vi "Actor Core.vi"(8 "error in":errorcluster, 11 "Example Controller":refnum<class "Example Controller.lvclass">) -> (0 "error out":errorcluster, 3 "Actor out":refnum<class "Actor.lvclass">)   [LabVIEW 2023, in "Example MVC Actors.lvlib" / "Example Controller.lvlib" / "Example Controller.lvclass"]
doc: "This is Actor Core.vi, the main message handling loop for Actors. An actor usually just sits in this loop and processes messages as they arrive. Any error returned by the message Do.vi call will stop the loop, with error code 43 as the cannonical signal to stop with no error sent to caller. Descendants may override that in Handle Error.vi."
uses:
  Example Controller.lvclass
  <vilib>/ActorFramework/Actor/Actor.lvclass
  Registered Views.ctl
  Controller/View Settings.ctl
  Example Controller.lvclass/Example Controller.ctl
  Controller/Controller.lvclass/Controller.ctl
  <vilib>/ActorFramework/Actor/Actor.lvclass/Actor.ctl
  <vilib>/ActorFramework/Message Enqueuer/Message Enqueuer.lvclass/Message Enqueuer.ctl
  Write Boolean Notifier.vi
  Controller/properties/Read Registered Views Event Ref.vi
  Controller/properties/Read View Settings Event Ref.vi
  <vilib>/ActorFramework/Message Enqueuer/Init from Existing Queue.vi
  <vilib>/ActorFramework/Message Enqueuer/Enqueue.vi
  <vilib>/ActorFramework/Stop Msg/Stop Msg.lvclass
  <vilib>/Utility/LVClass/Get LV Class Name.vi
  <resource>/AFDebug/Generate Trace for Message.vi
  <vilib>/ActorFramework/Message Priority Queue/Priority Enqueue.vi
  <vilib>/ActorFramework/Message Enqueuer/Message Enqueuer.lvclass
  Timed Loop Controller/Timed Loop Controller/Timed Loop Controller.lvclass
  Controller/Controller.lvclass
  Controller Messages/Read View Settings Msg/Read View Settings Msg.lvclass
  Controller Messages/Write View Settings Msg/Write View Settings Msg.lvclass
  <userlib>/_OpenG.lib/error/error.llb/openg_error.lvlib
  Example Controller Messages/Launch Feature Test View Msg/Launch Feature Test View Msg.lvclass
panel:
  in  "Launch  Feature Test View":bool
  in  "View Settings":T1
  in  "Write View Settings":bool
  in  "Read View Settings":bool
  out "View Settings Read":T1
  in  "View":T2
  out "Boolean Chart":i16(graph)
  in  "Stop Button":bool
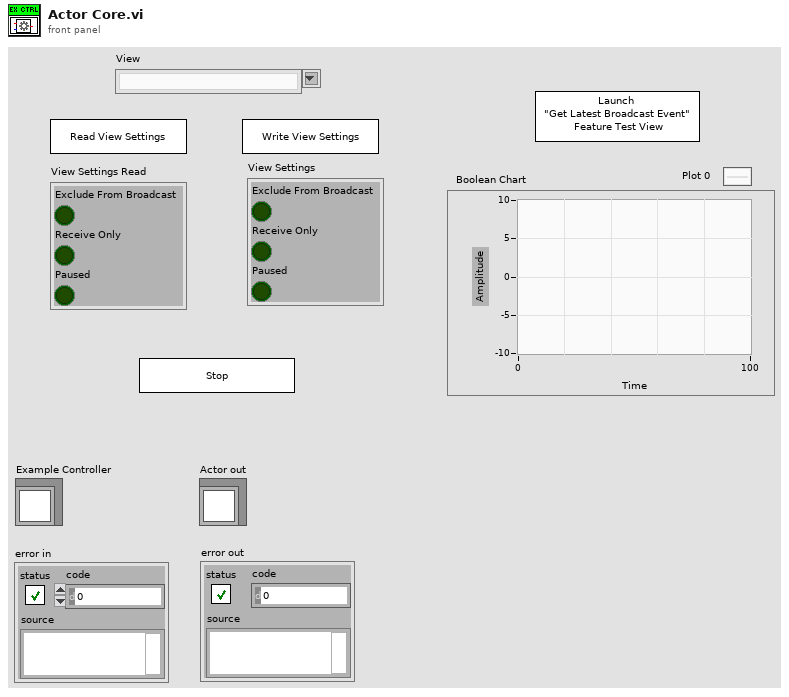
[diagram p1: front panel]
types:
  T1 = typedef "MVC Actors.lvlib/Controller.lvclass/View Settings.ctl" = cluster{"Exclude From Broadcast":bool, "Receive Only":bool, "Paused":bool}
  T2 = typedef "Example MVC Actors.lvlib/Example Controller.lvlib/Example Controller.lvclass/Registered Views.ctl" = string
  T3 = enum8{"Enabled", "Disabled", "Disabled and Grayed Out"}
  T4 = typedef "MVC Actors.lvlib/Controller.lvclass/Registered Views Event Ref.ctl" = refnum<user-event>
  T5 = typedef "MVC Actors.lvlib/Controller.lvclass/View Settings Event Ref.ctl" = refnum<user-event>
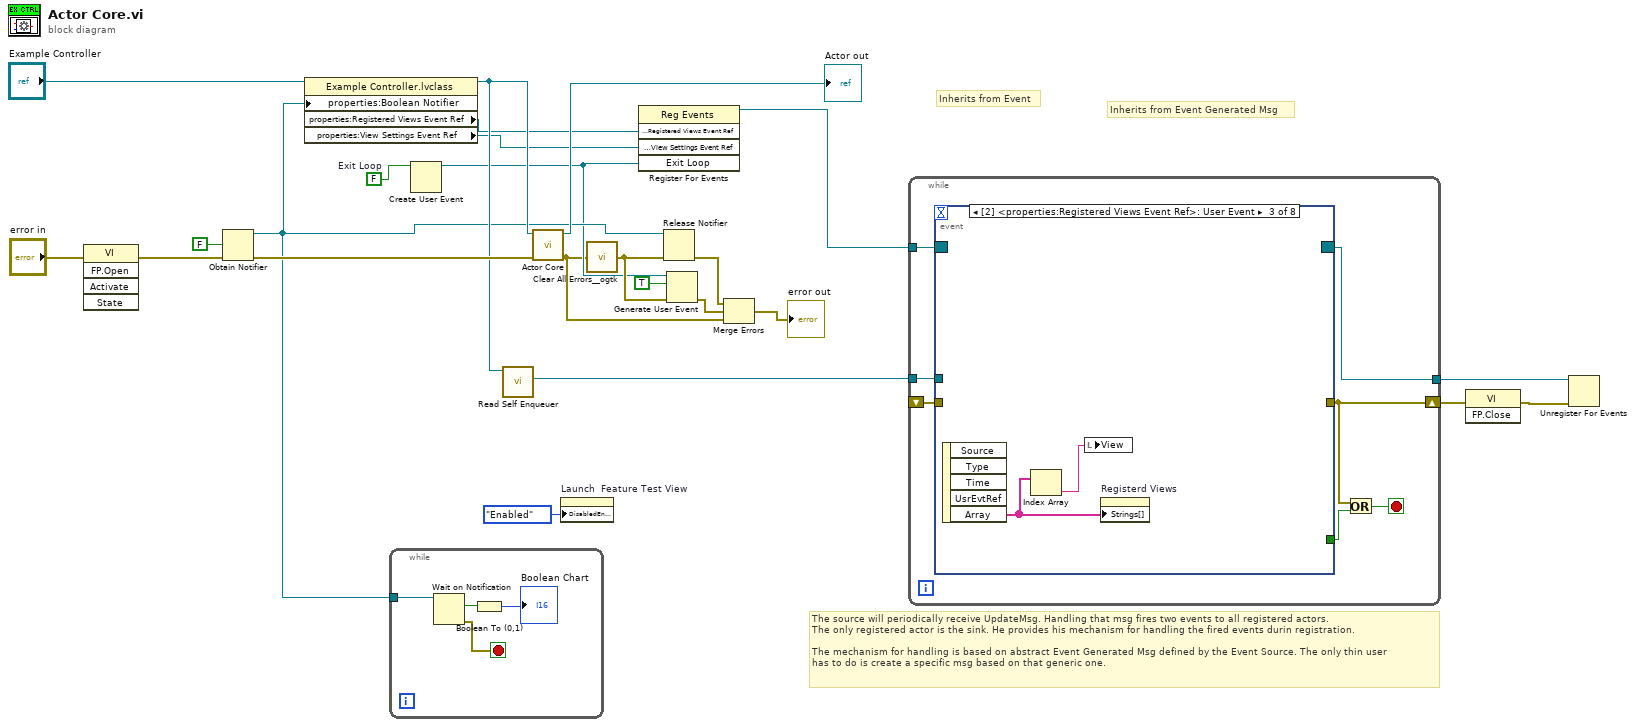
[diagram p0: block diagram]
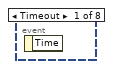
[diagram p2: hidden frame]
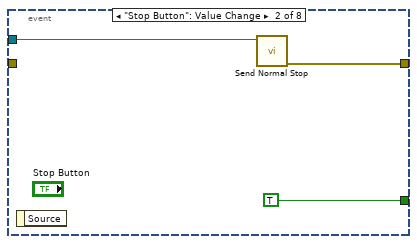
[diagram p3: hidden frame]
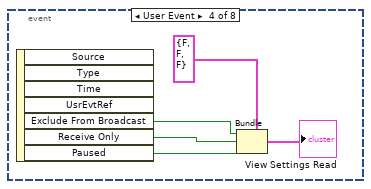
[diagram p4: hidden frame]
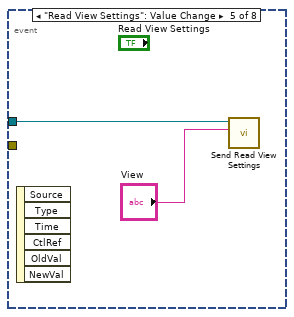
[diagram p5: hidden frame]
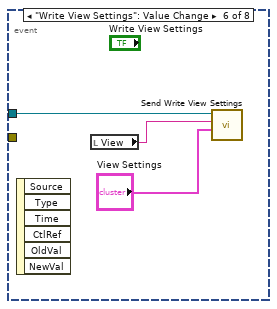
[diagram p6: hidden frame]
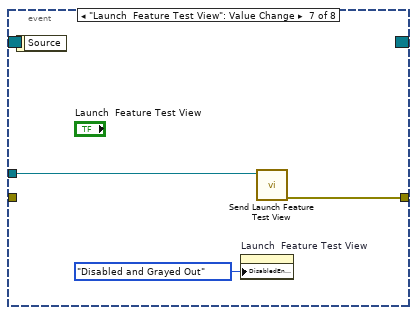
[diagram p7: hidden frame]
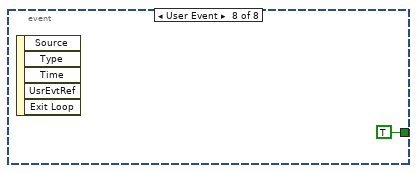
[diagram p8: hidden frame]
diagram:
  w11 = FALSE  # Exit Loop
  # "The source will periodically receive UpdateMsg. Handling that msg fires two events to all registered actors.\nThe only registered actor is the sink. He provides his mechanism for handling the fired events durin registration.\n\nThe mechanism for handling is based on abstract Event Generated Msg defined by the Event Source. The only thin user\nhas to do is create a specific msg based on that generic one."
  # "Inherits from Event"
  # "Inherits from Event Generated Msg"
  n1 = invoke on="Invoke Node" class="VI" method="FP.Open"(error in="error in") -> (error out=w2:errorcluster)  [unwired: 4 in, 4 out]
  n2 = Obtain Notifier(notification data type=FALSE, error in (no error)=w2) -> (notifier out=w18:refnum<notifier>, error out=w20:errorcluster)  [unwired: 2 in, 1 out]
  n3 = property class="Example Controller.lvclass"(reference="Example Controller", "properties:Boolean Notifier"=w18) -> (reference out=w19:refnum<class "Example Controller.lvclass">, "properties:Registered Views Event Ref"=w17:T4, "properties:View Settings Event Ref"=w16:T5)  [unwired: 1 in, 1 out]
  n4 = while {
    tunnel: w18 -> [w28]
    stop <- w25 stop-if-true
    n5 = Wait on Notification(notifier=w28) -> (notification=w27:bool, error out=w25:errorcluster)  [unwired: 3 in, 2 out]
    n6 = Boolean To (0,1)(Boolean=w27) -> (0, 1=→"Boolean Chart":i16)
  }
  n7 = Create User Event(user event datatype=w11) -> (user event=w8:refnum<user-event>)  [unwired: 1 in, 1 out]
  n8 = call <vilib>:"Read Self Enqueuer.vi"("Actor"=w19) -> ("Self Enqueuer"=w12:refnum<class "Message Enqueuer.lvclass">)  [unwired: 10 in]
  n9 = call-parent "Actor Core.vi"("error in"=w20, "Timed Loop Controller"=w19) -> ("error out"=w5:errorcluster, "Actor out"=→"Actor out":refnum<class "Actor.lvclass">)  [unwired: 8 in]
  n10 = property on="Launch  Feature Test View" class="Bool"("DisabledEnum"=T3."Enabled" ("Disabled")) -> ()  [unwired: 2 in, 2 out]
  n11 = call <userlib>:"Clear All Errors__ogtk.vi"("Error In"=w5) -> ("Error Out"=w9:errorcluster)  [unwired: 3 in]
  n12 = register-events(w17, w16, w8) -> (reference out=w15:refnum<event-registration>)  [unwired: 2 in, 1 out]
  n13 = Release Notifier(notifier=w18, error in (no error)=w9) -> (error out=w7:errorcluster)  [unwired: 1 in, 2 out]
  n14 = Generate User Event(user event=w8, event data cluster=TRUE ("event data"), error in=w9) -> (error out=w6:errorcluster)  [unwired: 1 in, 1 out]
  n15 = Merge Errors(w7, w6, w5) -> (→"error out":errorcluster)
  n16 = while {
    tunnel: w12 -> [w34]
    shift-right: [w32] -> w23
    shift-left: _ -> [w35]
    tunnel: w15 -> [w30]
    tunnel: [w29] -> w13
    stop <- w31 stop-if-true
    n17 = event shown="[2] <properties:Registered Views Event Ref>: User Event" {
      selector: w30 -> [_ _ _ _ _ _ _ _]
      dyn-events: [_ _ _ _ _ _ _ _] -> w29
      timeout: _ -> [_ _ _ _ _ _ _ _]
      tunnel: w35 -> [_ _ _ _ _ _ _ _]
      tunnel: w34 -> [_ w37 _ _ w46 w48 w53 _]
      tunnel: [_ w38 _ _ _ _ w52 _] -> w32
      tunnel: [_ TRUE _ _ _ _ _ TRUE] -> w33
      event Timeout {
        n18 = event-data() -> ()  [unwired: 1 in, 1 out]
      }
      event "Stop Button": Value Change {
        n19 = event-data() -> ()  [unwired: 1 in, 1 out]
        n20 = call <vilib>:"Send Normal Stop.vi"("Message Enqueuer"=w37) -> ("error out"=w38:errorcluster)  [unwired: 10 in]
      }
      event User Event {
        n21 = event-data() -> ("Array"=w40:string[])  [unwired: 1 in, 4 out]
        n22 = Index Array(array=w40) -> (element=w39:string)  [unwired: 1 in]
        n23 = local write "View"(w39) -> ()
        n24 = property on="Registerd Views" class="CmbBox (strict)"("Strings[]"=w40) -> ()  [unwired: 2 in, 2 out]
      }
      event User Event {
        n25 = event-data() -> ("Exclude From Broadcast"=w44:bool, "Receive Only"=w43:bool, "Paused"=w42:bool)  [unwired: 1 in, 4 out]
        n26 = Bundle(cluster=T1 {"Exclude From Broadcast"=FALSE, "Receive Only"=FALSE, "Paused"=FALSE} ("Sink Settings"), "Exclude From Broadcast"=w44, "Receive Only"=w43, "Paused"=w42) -> (→"View Settings Read":T1)
      }
      event "Read View Settings": Value Change {
        n27 = event-data() -> ()  [unwired: 1 in, 6 out]
        n28 = call "Send Read View Settings.vi"("View Name"="View", "Message Enqueuer in"=w46) -> ()  [unwired: 8 in, 2 out]
      }
      event "Write View Settings": Value Change {
        n29 = event-data() -> ()  [unwired: 1 in, 6 out]
        n30 = local read "View"() -> (w49:T2)
        n31 = call "Send Write View Settings.vi"("View Settings"="View Settings", "View Name"=w49, "Message Enqueuer in"=w48) -> ()  [unwired: 7 in, 2 out]
      }
      event "Launch  Feature Test View": Value Change {
        n32 = event-data() -> ()  [unwired: 1 in, 1 out]
        n33 = property on="Launch  Feature Test View" class="Bool"("DisabledEnum"=T3."Disabled and Grayed Out" ("Disabled")) -> ()  [unwired: 2 in, 2 out]
        n34 = call "Send Launch Feature Test View.vi"("Message Enqueuer in"=w53) -> ("error out"=w52:errorcluster)  [unwired: 9 in, 1 out]
      }
      event User Event {
        n35 = event-data() -> ()  [unwired: 1 in, 5 out]
      }
    }
    n36 = Or(x=w32, y=w33) -> (x .or. y?=w31:bool)
  }
  n37 = invoke class="VI" method="FP.Close"(error in=w23) -> (error out=w14:errorcluster)  [unwired: 2 in, 2 out]
  n38 = Unregister For Events(event registration refnum=w13, error in=w14) -> ()  [unwired: 1 out]
